vi "Get Product String.vi"(8 "error in (no error)":errorcluster, 9 "size":i32, 11 "index":i32) -> (0 "error out":errorcluster, 2 "string out":string, 3 "index_out":i32)   [LabVIEW 2013, in "FEMTO_LUCI-10.lvlib"]
doc: "This function reads the product string of the selected device."
uses:
  FEMTO_LUCI-10.lvlib
  LUCI_10.dll
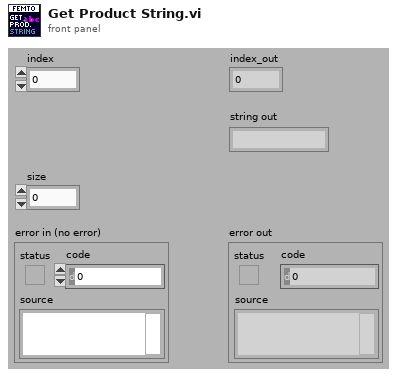
[diagram p1: front panel]
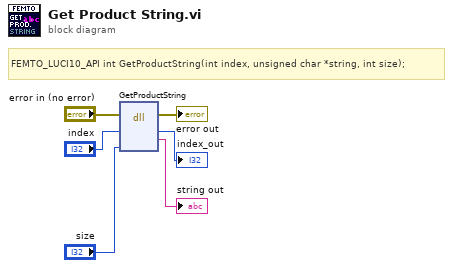
[diagram p0: block diagram]
diagram:
  # "FEMTO_LUCI10_API int GetProductString(int index, unsigned char *string, int size);"
  n1 = dll-call lib="C:/user/patrick/ppms_daq_femto/driver/LUCI_10.dll" fn="GetProductString"(error in="error in (no error)", "index"="index", "size"="size") -> (error out=→"error out":errorcluster, "index"=→"index_out":i32, "string"=→"string out":string)  [unwired: 3 in, 3 out]
